vi "connect data network stream.vi"(7 "Queues":T1, 11 "dataStream in":T2) -> (3 "dataStream out":T2)   [LabVIEW 2018]
uses:
  type defs/data stream data.ctl
  type defs/Queues.ctl
  supporting VIs/polymorphic VIs/enqueue for data stream.vi
  supporting VIs/polymorphic VIs/enqueue for message handler.vi
  RT/Message Handler loop/FPGA commands/RT - FPGA commands.lvlib
types:
  T1 = typedef "Queues.ctl" = cluster{"messageHandler":refnum<queue>, "comms":refnum<queue>, "dataStream":refnum<queue>, "dataProcessor":refnum<queue>, "fileIO":refnum<queue>, "userInterface":refnum<queue>, "errors":refnum<queue>, "customCompressor":refnum<queue>}
  T2 = typedef "data stream data.ctl" = cluster{"params":cluster{"Stream":cluster{"reader name":string, "RT IP address":string, "writer name":string, "stream buffer size":i32}}, "vars":cluster{"data stream":refnum<k21>}}
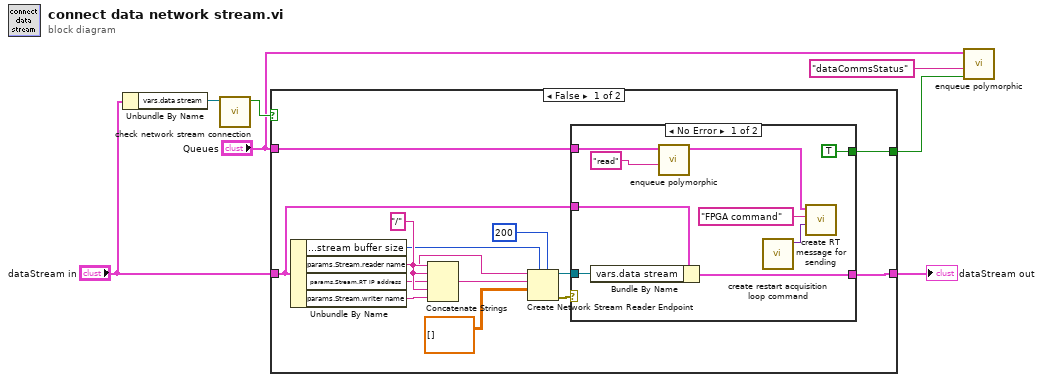
[diagram p0: block diagram]
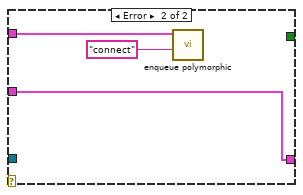
[diagram p2: hidden frame]
diagram:
  n1 = Unbundle By Name("dataStream in") -> ("vars.data stream"=w4:refnum<k21>)
  n2 = call "check network stream connection.vi"("stream ref"=w4) -> ("Connected"=w5:bool)  [unwired: 10 in]
  n3 = case shown="False" w5 {
    tunnel: [w21 w34] -> w7
    tunnel: "dataStream in" -> [w11 w34]
    tunnel: "Queues" -> [w8 _]
    tunnel: [w10 _] -> w2
    frame False {
      w18 = "/" ("string")
      n4 = Unbundle By Name(w11) -> ("params.Stream.stream buffer size"=w14:i32, "params.Stream.reader name"=w16:string, "params.Stream.RT IP address"=w17:string, "params.Stream.writer name"=w19:string)
      n5 = Concatenate Strings(w18, w18, w17, w18, w19) -> (w20:string)
      n6 = Create Network Stream Reader Endpoint(5:200 ("timeout in ms (-1)"), 7:w14, 9:dbl[][] [], 10:w20, 11:w16) -> (0:w12:errorcluster, 3:w9:refnum<k21>)  [unwired: 2 in]
      n7 = case shown="No Error" w12 {
        tunnel: w9 -> [w30 _]
        tunnel: [w29 w33] -> w21
        tunnel: w11 -> [w28 w33]
        tunnel: [TRUE _] -> w10
        tunnel: w8 -> [w25 w31]
        frame No Error {
          n8 = Bundle By Name(cluster=w28, "vars.data stream"=w30) -> (w29:T2)
          n9 = call-poly "enqueue polymorphic.vi"("message"="read", "Queues"=w25) -> ("Queues out"=w24:T1)  [unwired: 9 in]
          n10 = call "create restart acquisition loop command.vi"() -> ("command message"=w22:variant)  [unwired: 11 in]
          n11 = call "create RT message for sending.vi"("RT data"=w22, "RT message"="FPGA command" ("message"), "Queues in"=w24) -> ()  [unwired: 8 in, 1 out]
        }
        frame Error {
          n12 = call-poly "enqueue polymorphic.vi"("message"="connect", "Queues"=w31) -> ()  [unwired: 9 in, 1 out]
        }
      }
    }
    frame True {
    }
  }
  "dataStream out" <- w7
  n13 = call-poly "enqueue polymorphic.vi"("data"=w2, "message"="dataCommsStatus", "Queues"="Queues") -> ()  [unwired: 8 in, 1 out]
